vi "LoadClassDescriptionsByName.vi"(0 "Executer in":refnum<class "Executer.lvclass">, 1 "Class in":string, 5 "error in (no error)":errorcluster) -> (14 "Executer out":refnum<class "Executer.lvclass">, 15 "ClassDescription":T1, 19 "error out":errorcluster)   [LabVIEW 2018, in "Executer.lvclass"]
uses:
  Executer.lvclass
  typedefs/ClassDescription.ctl
  typedefs/MethodDescription.ctl
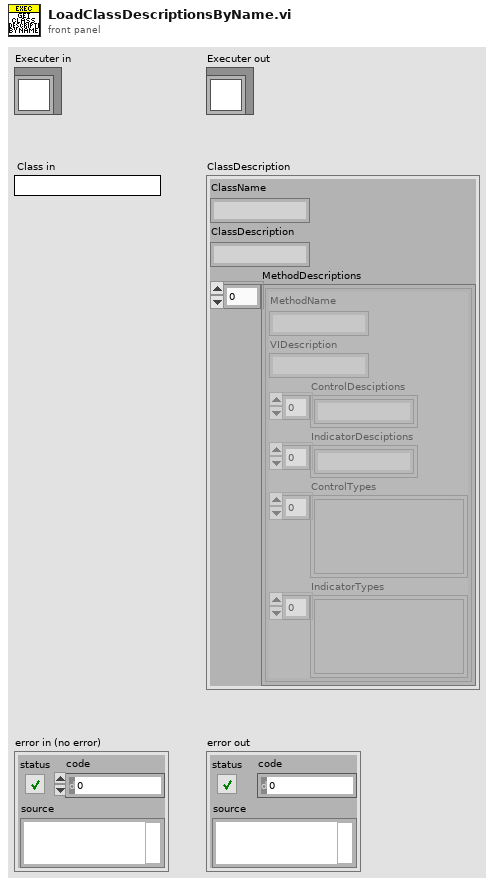
[diagram p1: front panel]
types:
  T1 = typedef "Executer.lvclass/ClassDescription.ctl" = cluster{"ClassName":string, "ClassDescription":string, "MethodDescriptions":T2[]}
  T2 = typedef "Executer.lvclass/MethodDescription.ctl" = cluster{"MethodName":string, "VIDescription":string, "ControlDesciptions":string[], "IndicatorDesciptions":string[], "ControlTypes":variant[], "IndicatorTypes":variant[]}
  T3 = typedef "Executer.lvclass/ObjectAttributes.ctl" = cluster{"Executions":T4[]}
  T4 = typedef "Executer.lvclass/ClassExecutionInfo.ctl" = cluster{"Class":refnum<class>, "ClassName":string, "VIExecutionInfo":T5[]}
  T5 = typedef "Executer.lvclass/MethodExecutionInfo.ctl" = cluster{"viRef":refnum<vi>, "MethodName":string, "ControlIndices":i32[], "ClassInIndex":i32, "IndicatorIndices":i32[], "ErrorOutIndex":i32, "ControlTypes":variant[]}
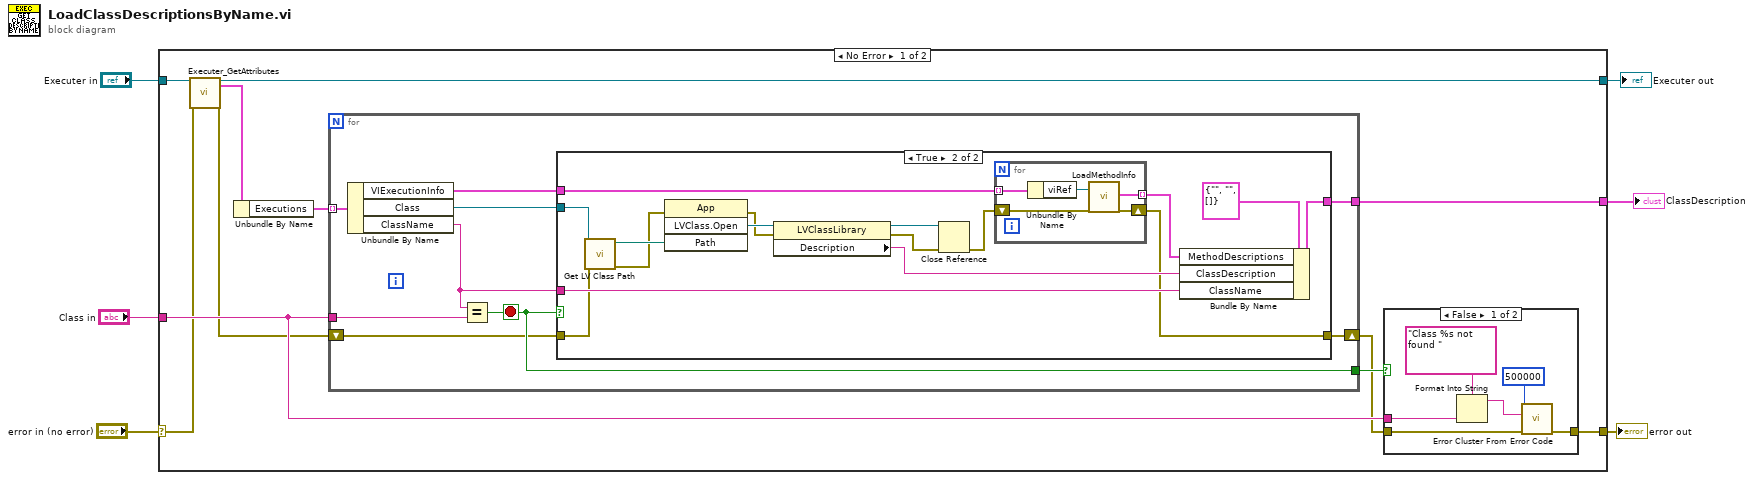
[diagram p0: block diagram]
diagram:
  n1 = case shown="No Error" "error in (no error)" {
    selector: "error in (no error)" -> [w11 w56]
    tunnel: [w16 w57] -> w6
    tunnel: "Executer in" -> [w15 w57]
    tunnel: "Class in" -> [w13 _]
    tunnel: [w12 w56] -> w4
    tunnel: [w7 _] -> w1
    frame No Error {
      n2 = call "Executer_GetAttributes.vi"("reference in"=w15, "error in (no error)"=w11) -> ("reference out"=w16:refnum<class "Executer.lvclass">, "Data"=w14:T3, "error out"=w9:errorcluster)  [unwired: 14 in, 1 out]
      n3 = Unbundle By Name(w14) -> ("Executions"=w17:T4[])
      n4 = for {
        tunnel: w17 -> [w25] mode=indexing
        tunnel: w13 -> [w26]
        tunnel: [w24] -> w10
        shift-right: [w20] -> w8
        shift-left: w9 -> [w21]
        tunnel: [w19] -> w7
        stop <- w24 stop-if-true
        n5 = Unbundle By Name(w25) -> ("VIExecutionInfo"=w18:T5[], "Class"=w22:refnum<class>, "ClassName"=w23:string)
        n6 = Equal?(x=w23, y=w26) -> (x = y?=w24:bool)
        n7 = case shown="True" w24 {
          tunnel: w23 -> [_ w37]
          tunnel: w22 -> [_ w38]
          tunnel: w18 -> [_ w36]
          tunnel: w21 -> [w27 w32]
          tunnel: [w27 w31] -> w20
          tunnel: [_ w30] -> w19
          frame False {
          }
          frame True {
            n8 = call <vilib>:"Get LV Class Path.vi"("error in (no error)"=w32, "object"=w38) -> ("error out"=w35:errorcluster, "class path"=w42:path)  [unwired: 8 in]
            n9 = invoke class="App" method="LVClass.Open"(error in=w35, "Path"=w42) -> (error out=w34:errorcluster, "LVClass.Open"=w43:refnum<vi>)  [unwired: 2 in, 2 out]
            n10 = property class="LVClassLibrary"(reference=w43, error in=w34) -> (reference out=w41:refnum<vi>, error out=w40:errorcluster, "Description"=w39:string)
            n11 = Close Reference(reference=w41, error in (no error)=w40) -> (error out=w33:errorcluster)
            n12 = for {
              tunnel: w36 -> [w48] mode=indexing
              tunnel: [w46] -> w28 mode=indexing
              shift-right: [w44] -> w31
              shift-left: w33 -> [w45]
              n13 = Unbundle By Name(w48) -> ("viRef"=w47:refnum<vi>)
              n14 = call "LoadMethodInfo.vi"("ViRef"=w47, "error in (no error)"=w45) -> ("Descriptions"=w46:T2, "error out"=w44:errorcluster)  [unwired: 15 in, 1 out]
            }
            n15 = Bundle By Name(cluster=T1 {"ClassName"="", "ClassDescription"="", "MethodDescriptions"=[]} ("ClassDescription"), "MethodDescriptions"=w28, "ClassDescription"=w39, "ClassName"=w37) -> (w30:T1)
          }
        }
      }
      n16 = case shown="False" w10 {
        tunnel: w13 -> [w51 _]
        tunnel: w8 -> [w50 w55]
        tunnel: [w49 w55] -> w12
        frame False {
          n17 = Format Into String(format string="Class %s not found ", w51) -> (resulting string=w53:string)  [unwired: 2 in, 1 out]
          n18 = call <vilib>:"Error Cluster From Error Code.vi"("error in (no error)"=w50, "error message (\"\")"=w53, "error code (0)"=500000) -> ("error out"=w49:errorcluster)  [unwired: 6 in]
        }
        frame True {
        }
      }
    }
    frame Error {
    }
  }
  "error out" <- w4
  "Executer out" <- w6
  "ClassDescription" <- w1
